vi "Write Boolean.vi"(8 "error in (no error)":errorcluster, 10 "Boolean":bool, 11 "NonBlueSerializable in":refnum<class "NonBlueSerializable.lvclass">) -> (0 "error out":errorcluster, 3 "NonBlueSerializable out":refnum<class "NonBlueSerializable.lvclass">)   [LabVIEW 2019, in "NonBlueSerializable.lvclass"]
uses:
  NonBlueSerializable.lvclass
  NonBlueSerializable.lvclass/NonBlueSerializable.ctl
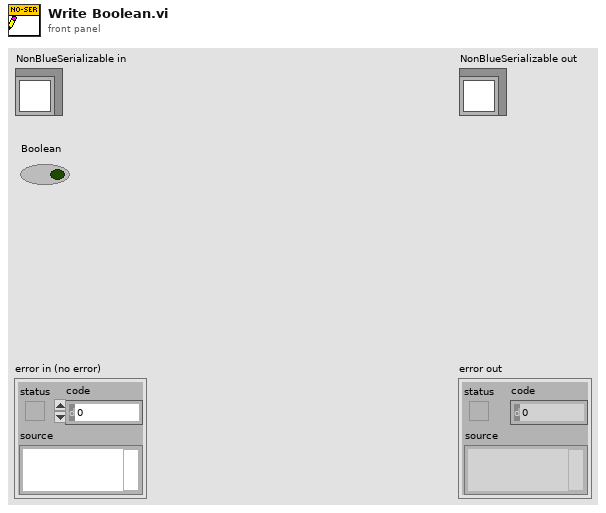
[diagram p1: front panel]
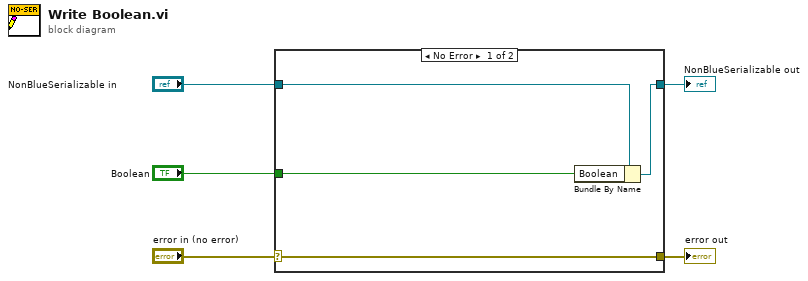
[diagram p0: block diagram]
diagram:
  n1 = case shown="No Error" "error in (no error)" {
    selector: "error in (no error)" -> [w9 w10]
    tunnel: [w9 w10] -> w4
    tunnel: [w7 w11] -> w2
    tunnel: "NonBlueSerializable in" -> [w8 w11]
    tunnel: "Boolean" -> [w6 _]
    frame No Error {
      n2 = Bundle By Name(cluster=w8, "Boolean"=w6) -> (w7:refnum<class "NonBlueSerializable.lvclass">)
    }
    frame Error {
    }
  }
  "error out" <- w4
  "NonBlueSerializable out" <- w2
